vi "Close Transport.vi"(8 "error in (no error)":errorcluster, 11 "ValueReferenceTransport in":refnum<class "ValueReferenceTransport.lvclass">) -> (0 "error out":errorcluster)   [LabVIEW 2015, in "Transport.lvlib" / "ValueReferenceTransport.lvclass"]
uses:
  ValueReferenceTransport.lvclass
  ValueReferenceTransport.lvclass/ValueReferenceTransport.ctl
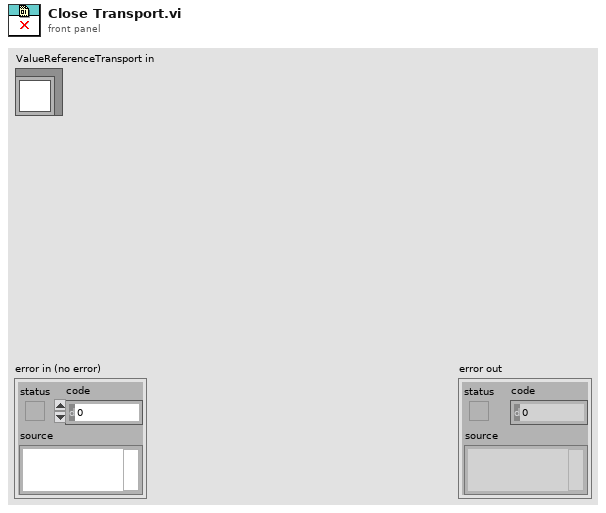
[diagram p1: front panel]
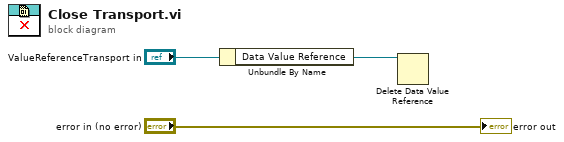
[diagram p0: block diagram]
diagram:
  n1 = Unbundle By Name("ValueReferenceTransport in") -> ("Data Value Reference"=w1:refnum<data-value>)
  n2 = Delete Data Value Reference(data value reference=w1) -> ()  [unwired: 1 in, 2 out]
  "error out" <- "error in (no error)"
